vi "test Add-Find-Remove.vi"(8 "error in (no error)":errorcluster, 11 "TestCase in":refnum<class "Scripting.lvclass">) -> (0 "error out":errorcluster, 3 "TestCase out":refnum<class "Scripting.lvclass">)   [LabVIEW 2020, in "Scripting.lvclass"]
uses:
  Scripting.lvclass
  <vilib>/addons/_JKI Toolkits/VI Tester/TestCase.llb/TestCase.lvclass
  Scripting/Communication Bus Template Scripting.lvlib
  C:/Program Files (x86)/National Instruments/LabVIEW 2020/vi.lib/addons/_JKI Toolkits/VI Tester/TestCase.llb/TestCase.lvclass
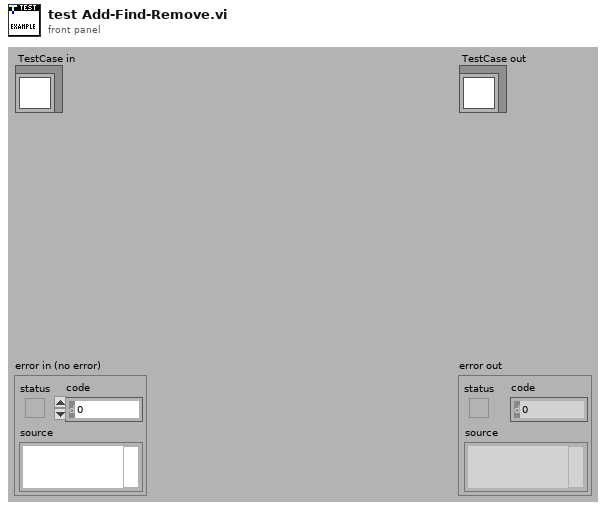
[diagram p1: front panel]
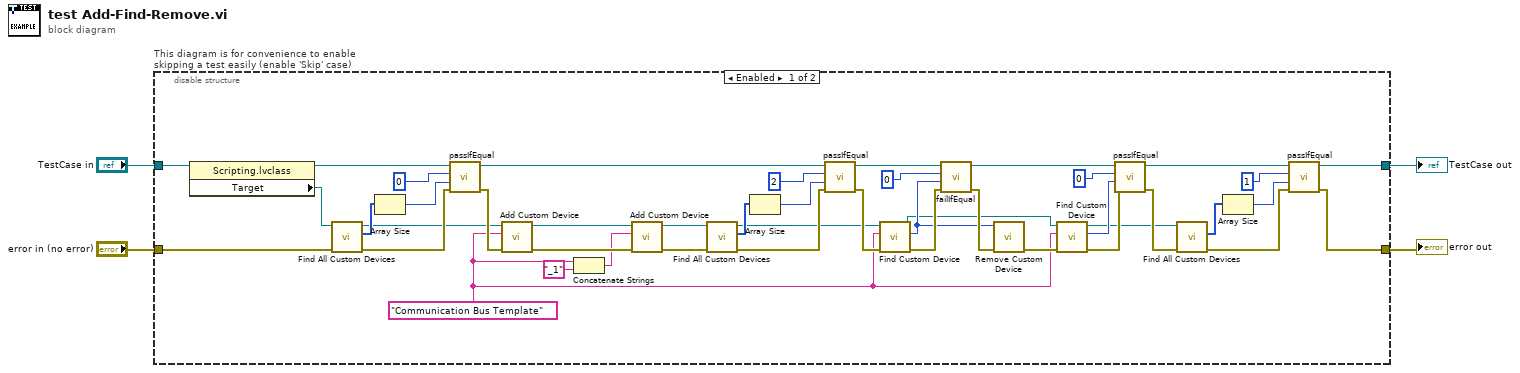
[diagram p0: block diagram]
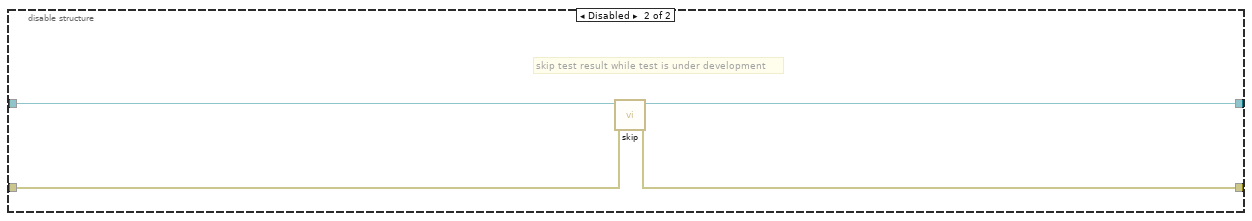
[diagram p2: hidden frame]
diagram:
  n1 = disable-structure "This diagram is for convenience to enable skipping a test easily (enable 'Skip' case)" shown="Enabled" {
    disable-tunnel: "TestCase in" -> [w5 w52]
    disable-tunnel: [w6 w50] -> w1
    disable-tunnel: [w7 w51] -> w3
    disable-tunnel: "error in (no error)" -> [w8 w49]
    frame Enabled {
      w24 = "Communication Bus Template" ("name")
      n2 = property class="Scripting.lvclass"(reference=w5) -> (reference out=w9:refnum<class "Scripting.lvclass">, "Target"=w10:refnum<k24>)  [unwired: 1 in, 1 out]
      n3 = call "Find All Custom Devices.vi"("error in"=w8, "target in"=w10) -> ("error out"=w45:errorcluster, "custom devices"=w48:u64[], "target out"=w43:refnum<k24>)  [unwired: 7 in]
      n4 = Array Size(array=w48) -> (size(s)=w47:i32)
      n5 = call-dynamic "passIfEqual.vi"("error in (no error)"=w45, "y"=w47, "x"=0 ("size(s)"), "TestCase in"=w9) -> ("error out"=w44:errorcluster, "TestCase out"=w33:refnum<class "Scripting.lvclass">)  [unwired: 6 in]
      n6 = call "Add Custom Device.vi"("error in"=w44, "name"=w24, "target in"=w43) -> ("error out"=w41:errorcluster, "target out"=w40:refnum<k24>)  [unwired: 6 in, 1 out]
      n7 = Concatenate Strings(w24, "_1" ("string")) -> (w39:string)
      n8 = call "Add Custom Device.vi"("error in"=w41, "name"=w39, "target in"=w40) -> ("error out"=w38:errorcluster, "target out"=w37:refnum<k24>)  [unwired: 6 in, 1 out]
      n9 = call "Find All Custom Devices.vi"("error in"=w38, "target in"=w37) -> ("error out"=w32:errorcluster, "custom devices"=w34:u64[], "target out"=w30:refnum<k24>)  [unwired: 7 in]
      n10 = Array Size(array=w34) -> (size(s)=w35:i32)
      n11 = call-dynamic "passIfEqual.vi"("error in (no error)"=w32, "y"=w35, "x"=2 ("size(s)"), "TestCase in"=w33) -> ("error out"=w31:errorcluster, "TestCase out"=w29:refnum<class "Scripting.lvclass">)  [unwired: 6 in]
      n12 = call "Find Custom Device.vi"("error in"=w31, "name"=w24, "target in"=w30) -> ("error out"=w28:errorcluster, "custom device"=w26:u64, "target out"=w23:refnum<k24>)  [unwired: 6 in]
      n13 = call-dynamic "failIfEqual.vi"("error in (no error)"=w28, "y"=w26, "x"=u64 0 ("custom device"), "TestCase in"=w29) -> ("error out"=w27:errorcluster, "TestCase out"=w22:refnum<class "Scripting.lvclass">)  [unwired: 6 in]
      n14 = call "Remove Custom Device.vi"("error in"=w27, "custom device"=w26) -> ("error out"=w25:errorcluster)  [unwired: 9 in]
      n15 = call "Find Custom Device.vi"("error in"=w25, "name"=w24, "target in"=w23) -> ("error out"=w18:errorcluster, "custom device"=w20:u64, "target out"=w16:refnum<k24>)  [unwired: 6 in]
      n16 = call-dynamic "passIfEqual.vi"("error in (no error)"=w18, "y"=w20, "x"=u64 0 ("custom device"), "TestCase in"=w22) -> ("error out"=w17:errorcluster, "TestCase out"=w14:refnum<class "Scripting.lvclass">)  [unwired: 6 in]
      n17 = call "Find All Custom Devices.vi"("error in"=w17, "target in"=w16) -> ("error out"=w13:errorcluster, "custom devices"=w12:u64[])  [unwired: 7 in, 1 out]
      n18 = Array Size(array=w12) -> (size(s)=w11:i32)
      n19 = call-dynamic "passIfEqual.vi"("error in (no error)"=w13, "y"=w11, "x"=1 ("size(s)"), "TestCase in"=w14) -> ("error out"=w7:errorcluster, "TestCase out"=w6:refnum<class "Scripting.lvclass">)  [unwired: 6 in]
    }
    frame Disabled {
      # "skip test result while test is under development"
      n20 = call <vilib>:"skip.vi"("error in (no error)"=w49, "TestCase in"=w52) -> ("error out"=w51:errorcluster, "TestCase out"=w50:refnum<class "Scripting.lvclass">)  [unwired: 8 in]
    }
  }
  "error out" <- w3
  "TestCase out" <- w1
